vi "SEQ Preview Queue.vi"(8 "error in (no error)":errorcluster, 11 "Queue Name":string) -> (0 "error out":errorcluster, 2 "Setting":T1)   [LabVIEW 2019, in "ADLINK Motion Card.lvlib"]
uses:
  ADLINK Motion Card.lvlib
  SEQ Data.ctl
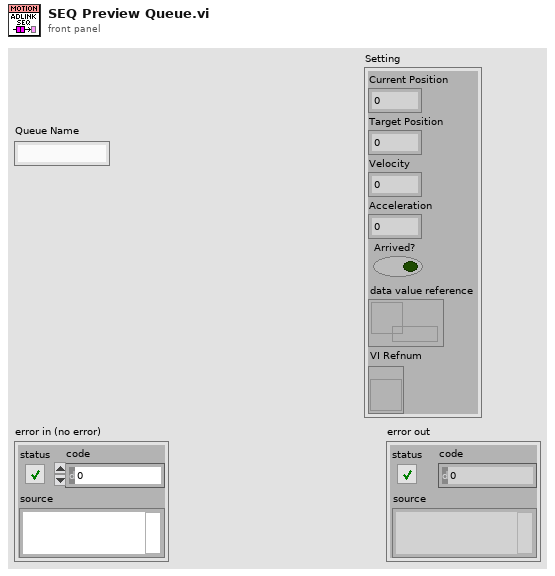
[diagram p1: front panel]
types:
  T1 = typedef "ADLINK Motion Card.lvlib/SEQ Data.ctl" = cluster{"Current Position":dbl, "Target Position":dbl, "Velocity":dbl, "Acceleration":dbl, "Arrived?":bool, "data value reference":refnum<data-value>, "VI Refnum":refnum<vi>}
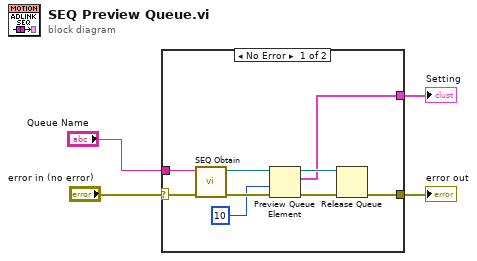
[diagram p0: block diagram]
diagram:
  n1 = case shown="No Error" "error in (no error)" {
    selector: "error in (no error)" -> [w8 w14]
    tunnel: "Queue Name" -> [w13 _]
    tunnel: [w6 _] -> w3
    tunnel: [w7 w14] -> w1
    frame No Error {
      n2 = call "SEQ Obtain.vi"("error in (no error)"=w8, "Queue Name"=w13) -> ("error out"=w11:errorcluster, "queue out"=w12:refnum<queue>)  [unwired: 8 in]
      n3 = Preview Queue Element(queue=w12, timeout in ms (-1)=10, error in (no error)=w11) -> (queue out=w10:refnum<queue>, element=w6:T1, error out=w9:errorcluster)  [unwired: 1 out]
      n4 = Release Queue(queue=w10, error in (no error)=w9) -> (error out=w7:errorcluster)  [unwired: 1 in, 2 out]
    }
    frame Error {
    }
  }
  "error out" <- w1
  "Setting" <- w3
